vi "Cleanup.vi"(8 "error in (no error)":errorcluster, 11 "InsertionPalettePanel in":refnum<class "InsertionPalettePanel.lvclass">) -> (0 "error out":errorcluster)   [LabVIEW 2020, in "TSnax UI.lvlib" / "InsertionPalettePanel.lvclass"]
uses:
  InsertionPalettePanel.lvclass
  InsertionPalettePanel.lvclass/InsertionPalettePanel.ctl
  <vilib>/IlluminatedG/IG OOPanel/OOPanel/Panel/Panel.lvclass
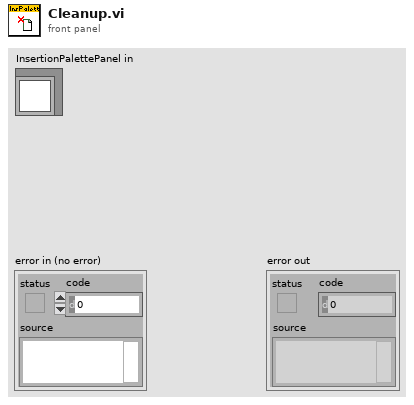
[diagram p1: front panel]
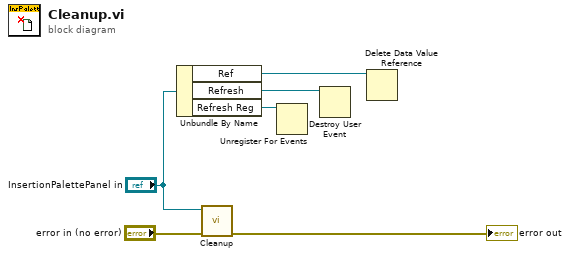
[diagram p0: block diagram]
diagram:
  n1 = Unbundle By Name("InsertionPalettePanel in") -> ("Ref"=w1:refnum<data-value>, "Refresh"=w2:refnum<user-event>, "Refresh Reg"=w3:refnum<event-registration>)
  n2 = call-parent "Cleanup.vi"("error in (no error)"="error in (no error)", "Panel in"="InsertionPalettePanel in") -> ("error out"=→"error out":errorcluster)  [unwired: 9 in]
  n3 = Unregister For Events(event registration refnum=w3) -> ()  [unwired: 1 in, 1 out]
  n4 = Destroy User Event(user event=w2) -> ()  [unwired: 1 in, 1 out]
  n5 = Delete Data Value Reference(data value reference=w1) -> ()  [unwired: 1 in, 2 out]
